vi "Configuration File--constant.vi"() -> (3 "Configuration File":refnum<class "Peloton_DCFG File.lvclass">)   [LabVIEW 2020, in "Rename As Application UI.lvlib" / "Configuration.lvlib"]
doc: "This VI stores the path at which the configuration file is stored, saved in a configuration file object.\n_____\nBased on DCFG Project Template 1.0.0.21.\n____\nPeloton Config 1.0.0.2\nCopyright (c) 2022, Peloton"
uses:
  Configuration.lvlib
  <vilib>/Peloton/Peloton Config/Libraries/DCFG File_class/Peloton_DCFG File.lvclass
  <vilib>/Peloton/Peloton Config/Libraries/DCFG File_class/Peloton_DCFG File.lvclass/Peloton_DCFG File.ctl
  <vilib>/Peloton/Peloton Config/Libraries/DCFG File_class/Set File Path.vi
  <vilib>/Peloton/Peloton Config/Libraries/DCFG Framework/Peloton_DCFG Framework.lvlib
panel:
  out "Configuration Path":path
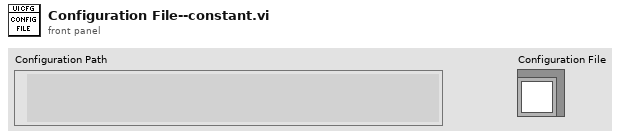
[diagram p1: front panel]
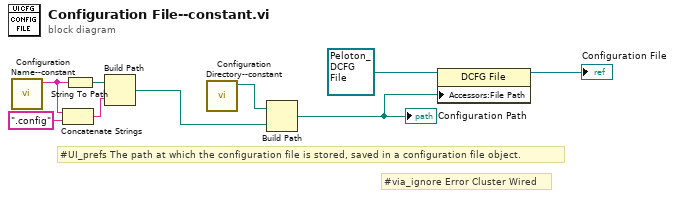
[diagram p0: block diagram]
diagram:
  # "#via_ignore Error Cluster Wired"
  # "#UI_prefs The path at which the configuration file is stored, saved in a configuration file object."
  n1 = call "Configuration Name--constant.vi"() -> ("Configuration Name"=w4:string)  [unwired: 11 in]
  n2 = Concatenate Strings(w4, ".config" ("string")) -> (w2:string)
  n3 = String To Path(string=w4) -> (path=w5:path)
  n4 = Build Path(base path=w5, name or relative path=w2) -> (appended path=w1:path)
  n5 = call <vilib>:"Configuration Directory--constant.vi"() -> ("CFG Directory"=w9:path)  [unwired: 11 in]
  n6 = Build Path(base path=w9, name or relative path=w1) -> (appended path=w6:path)
  "Configuration Path" <- w6
  n7 = property class="DCFG File"(reference=refnum<class "Peloton_DCFG File.lvclass"> refnum ("Configuration File"), "Accessors:File Path"=w6) -> (reference out=→"Configuration File":refnum<class "Peloton_DCFG File.lvclass">)  [unwired: 1 in, 1 out]
